vi "create.vi"(8 "error in (no error)":errorcluster) -> (0 "error out":errorcluster, 3 "Credit Transactions out":refnum<class "CreditTransactionList.lvclass">)   [LabVIEW 2018, in "CreditTransactionList.lvclass"]
uses:
  CreditTransactionList.lvclass
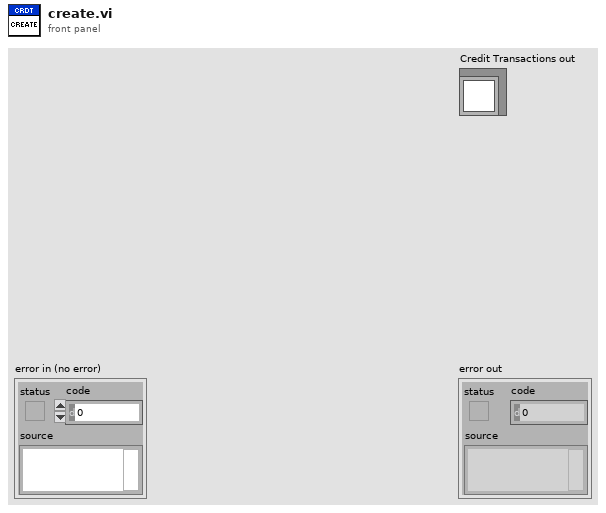
[diagram p1: front panel]
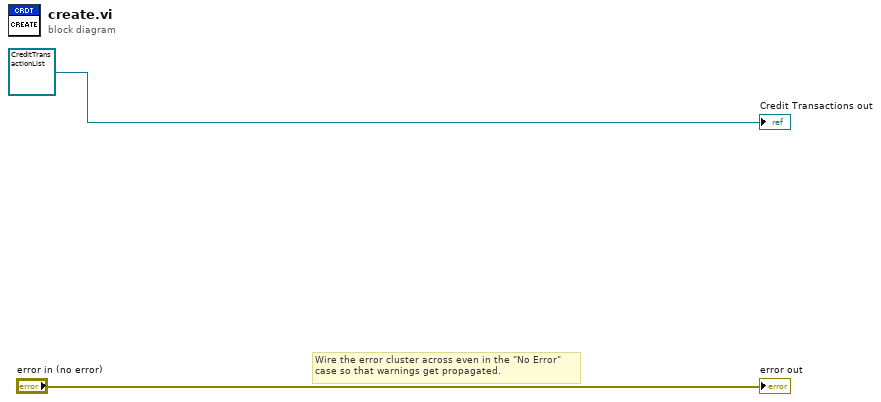
[diagram p0: block diagram]
diagram:
  # "Wire the error cluster across even in the \"No Error\"\ncase so that warnings get propagated."
  "error out" <- "error in (no error)"
  "Credit Transactions out" <- refnum<class "CreditTransactionList.lvclass"> refnum ("Credit Transactions in")
